vi "Read Binary Recovery File.vi"(8 "error in":errorcluster, 11 "File Path":path) -> (0 "error out":errorcluster, 2 "Data Out":dbl[][](array[numeric]) format="%0.2f")   [LabVIEW 2021]
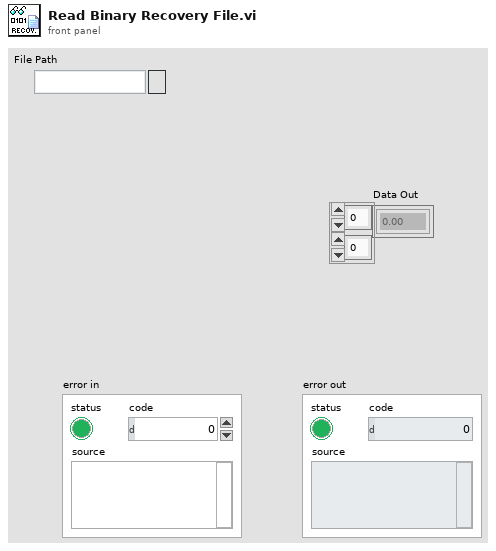
[diagram p1: front panel]
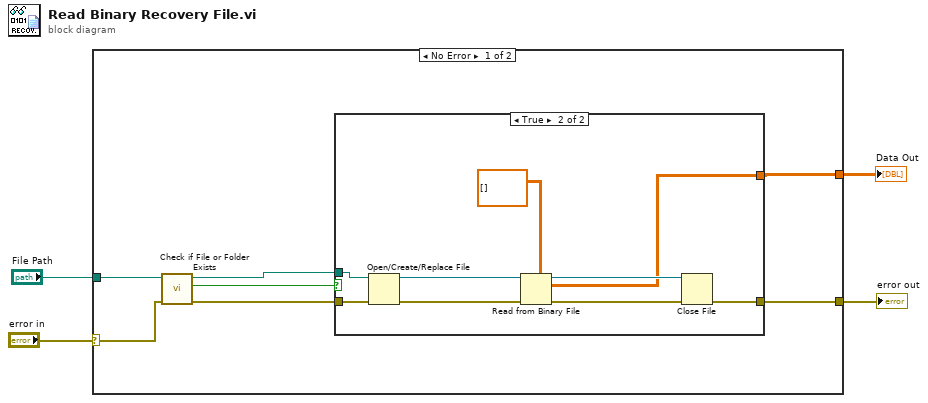
[diagram p0: block diagram]
diagram:
  n1 = case shown="No Error" "error in" {
    selector: "error in" -> [w9 w22]
    tunnel: "File Path" -> [w10 _]
    tunnel: [w6 w22] -> w2
    tunnel: [w5 _] -> w1
    frame No Error {
      n2 = call <vilib>:"Check if File or Folder Exists.vi"("error in (no error)"=w9, "path"=w10) -> ("error out"=w8:errorcluster, "file or folder exists?"=w11:bool, "dup path"=w7:path)  [unwired: 7 in]
      n3 = case shown="True" w11 {
        tunnel: w8 -> [w12 w21]
        tunnel: w7 -> [_ w16]
        tunnel: [w12 w18] -> w6
        tunnel: [_ w13] -> w5
        frame False {
        }
        frame True {
          n4 = Open/Create/Replace File(file path (use dialog)=w16, error in=w21) -> (refnum out=w15:refnum<file>, error out=w20:errorcluster)  [unwired: 4 in, 1 out]
          n5 = Read from Binary File(5:dbl[][] [] ("Data Out"), 8:w20, 11:w15) -> (0:w19:errorcluster, 2:w13:dbl[][], 3:w14:refnum<file>)  [unwired: 3 in, 1 out]
          n6 = Close File(refnum=w14, error in=w19) -> (error out=w18:errorcluster)  [unwired: 1 out]
        }
      }
    }
    frame Error {
    }
  }
  "Data Out" <- w1
  "error out" <- w2
